vi "Poll.RateProperties.vi"(7 "Action":enum8{"Get", "Set"}(ring), 8 "error in (no error)":errorcluster, 10 "Poll Rate":dbl=100.0, 11 "Item Ref in":T1 format="%.0x") -> (0 "error out":errorcluster, 2 "Poll Rate":dbl, 3 "Item Ref out":T1 format="%.0x")   [LabVIEW 2015, in "OPC UA Client System Explorer.lvlib"]
uses:
  OPC UA Client System Explorer.lvlib
  <vilib>/NI Veristand/Custom Device API/Custom Device Item Ref.ctl
  Shared/Constants.vi
  <vilib>/NI Veristand/Custom Device API/Get Item Property (Double).vi
  <vilib>/NI Veristand/Custom Device API/Set Item Property (Double).vi
  <vilib>/NI VeriStand/Custom Device API/Custom Device API.lvlib
  Shared/OPC UA Client Shared.lvlib
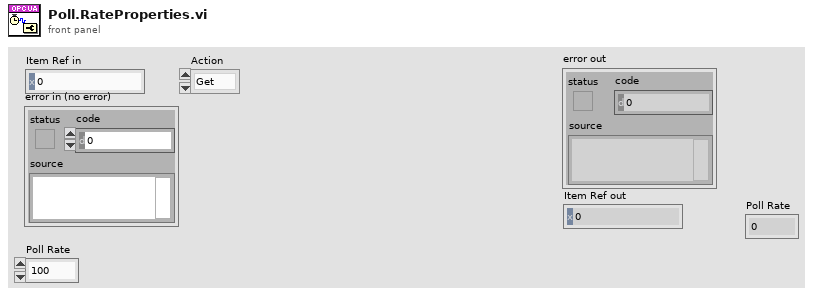
[diagram p1: front panel]
types:
  T1 = typedef "Custom Device API.lvlib/Custom Device Item Ref.ctl" = u64
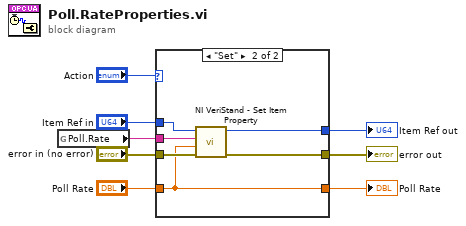
[diagram p0: block diagram]
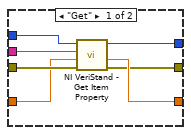
[diagram p2: hidden frame]
diagram:
  n1 = global read "Constants.vi" "Poll.Rate"() -> (w8:string)
  n2 = case shown="\"Set\"" "Action" {
    tunnel: w8 -> [w13 w21]
    tunnel: [w10 w17] -> w7
    tunnel: [w9 w16] -> w6
    tunnel: "Item Ref in" -> [w14 w20]
    tunnel: "error in (no error)" -> [w15 w19]
    tunnel: "Poll Rate" -> [w12 w18]
    tunnel: [w11 w18] -> w2
    frame "Get" {
      n3 = call-poly <vilib>:"NI VeriStand - Get Item Property.vi"("error in (no error)"=w15, "Default Value"=w12, "Property Name"=w13, "Item Ref in"=w14) -> ("error out"=w10:errorcluster, "Value"=w11:dbl, "Item Ref out"=w9:T1)  [unwired: 4 in, 1 out]
    }
    frame "Set" {
      n4 = call-poly <vilib>:"NI VeriStand - Set Item Property.vi"("error in (no error)"=w19, "Value"=w18, "Property Name"=w21, "Item Ref in"=w20) -> ("error out"=w17:errorcluster, "Item Ref out"=w16:T1)  [unwired: 5 in, 1 out]
    }
  }
  "error out" <- w7
  "Item Ref out" <- w6
  "Poll Rate" <- w2
